vi "Dev Fetch.vi"(8 "error in (no error)":errorcluster, 9 "firmware revision":string(combo), 10 "dev point (ALL)":u16(ring)=2 items=["CAP", "LOSS", "ALL"], 11 "VISA resource name":refnum<visa-resource-name>) -> (0 "error out":errorcluster, 2 "bridge error":T1, 3 "VISA resource name out":refnum<visa-resource-name>)   [LabVIEW 2024, in "Andeen-Hagerling 2700A.lvlib"]
doc: "Sets the capacitance and/or the loss values for the Deviation Setpoint to the most recent bridge mode measurement value."
uses:
  Andeen-Hagerling 2700A.lvlib
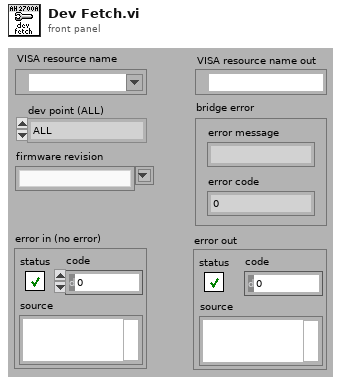
[diagram p1: front panel]
types:
  T1 = cluster{"error message":string, "error code":i32}
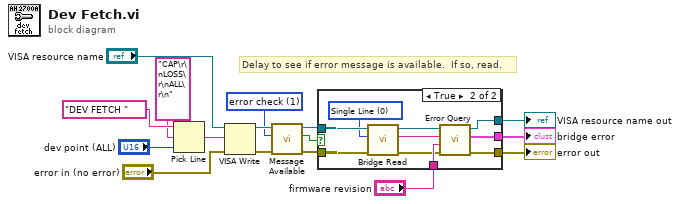
[diagram p0: block diagram]
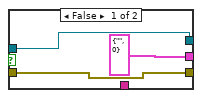
[diagram p2: hidden frame]
diagram:
  w1 = u16 1 items=["none", "error check", "multiline read", "infinite"] ("delay")
  # "Delay to see if error message is available.  If so, read."
  n1 = Pick Line(string ("")="DEV FETCH " ("command"), multi-line string="CAP\r\nLOSS\r\nALL\r\n" ("options"), line index="dev point (ALL)") -> (output string=w12:string)
  n2 = VISA Write(VISA resource name="VISA resource name", write buffer=w12, error in (no error)="error in (no error)") -> (VISA resource name out=w6:refnum<visa-resource-name>, error out=w5:errorcluster)  [unwired: 1 out]
  n3 = call "Message Available.vi"("error in (no error)"=w5, "delay"=w1, "VISA resource name"=w6) -> ("error out"=w8:errorcluster, "message available"=w10:bool, "VISA resource name out"=w9:refnum<visa-resource-name>)  [unwired: 6 in]
  n4 = case shown="True" w10 {
    tunnel: w9 -> [w18 w25]
    tunnel: w8 -> [w19 w24]
    tunnel: "firmware revision" -> [_ w29]
    tunnel: [w19 w28] -> w4
    tunnel: [w18 w27] -> w3
    tunnel: [T1 {"error message"="", "error code"=0} ("bridge error") w26] -> w2
    frame False {
    }
    frame True {
      w20 = u16 0 items=["Single Line", "Multi-Line"] ("Multiline")
      n5 = call "Bridge Read.vi"("error in (no error)"=w24, "multiline"=w20, "VISA resource name"=w25) -> ("error out"=w21:errorcluster, "read buffer"=w22:string, "VISA resource name out"=w23:refnum<visa-resource-name>)  [unwired: 6 in]
      n6 = call "Error Query.vi"("error in (no error)"=w21, "firmware revision"=w29, "measurement line"=w22, "VISA resource name"=w23) -> ("error out"=w28:errorcluster, "bridge error"=w26:T1, "VISA resource name out"=w27:refnum<visa-resource-name>)  [unwired: 5 in]
    }
  }
  "VISA resource name out" <- w3
  "error out" <- w4
  "bridge error" <- w2
